vi "ToBackMap-V2.2.vi"(4 "Column":i32, 5 "Row":i32, 6 "BackMap":i32[][](array[numeric])) -> (1 "String":string, 2 "Numeric":dbl)   [LabVIEW 2014]
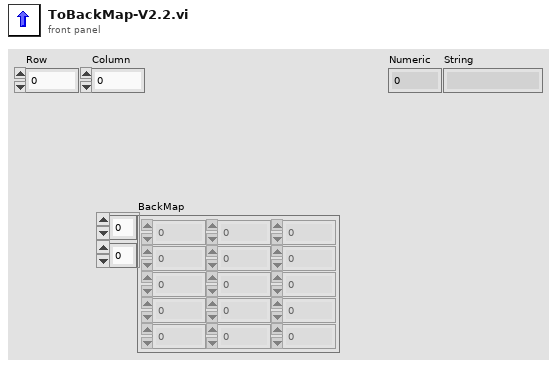
[diagram p1: front panel]
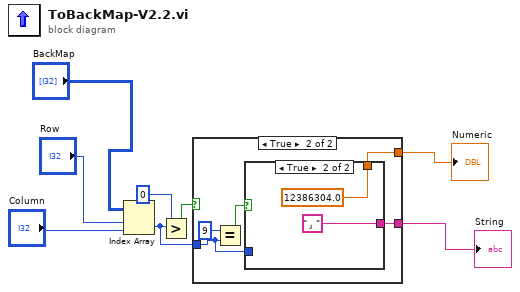
[diagram p0: block diagram]
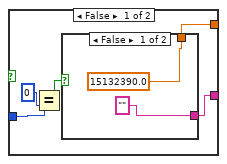
[diagram p2: hidden frame]
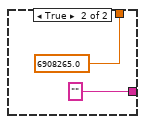
[diagram p3: hidden frame]
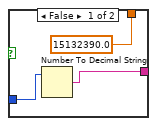
[diagram p4: hidden frame]
diagram:
  n1 = Index Array(array="BackMap", index (row)="Row", index (col)="Column") -> (element=w6:i32)
  n2 = Greater?(x=w6, y=0) -> (0:w7:bool)
  n3 = case shown="True" w7 {
    tunnel: [w9 w22] -> w2
    tunnel: [w10 w21] -> w1
    tunnel: w6 -> [w13 w18]
    frame False {
      n4 = Equal?(x=w13, y=0) -> (x = y?=w11:bool)
      n5 = case shown="False" w11 {
        tunnel: ["" ""] -> w10
        tunnel: [15132390.0 6908265.0] -> w9
        frame False {
        }
        frame True {
        }
      }
    }
    frame True {
      n6 = Equal?(x=9, y=w18) -> (x = y?=w19:bool)
      n7 = case shown="True" w19 {
        tunnel: [15132390.0 12386304.0] -> w22
        tunnel: [w24 "」"] -> w21
        tunnel: w18 -> [w25 _]
        frame False {
          n8 = Number To Decimal String(number=w25) -> (decimal integer string=w24:string)  [unwired: 1 in]
        }
        frame True {
        }
      }
    }
  }
  "Numeric" <- w2
  "String" <- w1
